vi "Untitled 6.vi"() -> ()   [LabVIEW 2016]
panel:
  in  "Stimulus parameters":T1={"Name"="", "Active bottles"=[3, 6], "Concentrations"=[1.0], "Unit"=enum."ppm", "Pulse duration (ms)"=250.0}
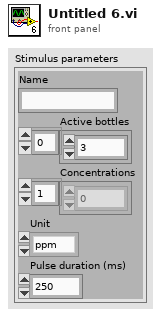
[diagram p1: front panel]
types:
  T1 = cluster{"Name":string, "Active bottles":i32[], "Concentrations":dbl[], "Unit":enum16{"%", "ppm"}, "Pulse duration (ms)":dbl}
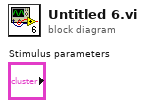
[diagram p0: block diagram]
diagram:
